vi "PatchCore_DS_Reader_old.vi"(4 "Read Bads?":bool, 5 "Input3D_Custom_Dims":T1, 6 "PreProcessing_Options":T2={"Image Type"=4, "Normalization Type"=enum."Standardize(DS_Stats)", "Interpolation Type"=1} {"Interpolation Type" items=["Zero Order", "Bi-Linear", "Quadratic", "Cubic Spline"]; "Image Type" items=["Grayscale (U8)", "Grayscale (I16)", "Grayscale (SGL)", "Complex (CSG)", "RGB (U32)", "HSL (U32)", "RGB (U64)", "Grayscale (U16)"]}, 7 "Dataset_Stats":T8={"means"={"R"=0.30100304, "G"=0.3015279, "B"=0.32350188}, "vars"={"R"=0.30371806, "G"=0.30376178, "B"=0.2861995}, "DS_Size"=0} {"vars"."R" format="%#_3g"; "vars"."G" format="%#_3g"; "vars"."B" format="%#_3g"; "means"."R" format="%#_3g"; "means"."G" format="%#_3g"; "means"."B" format="%#_3g"}, 8 "error in":errorcluster, 9 "GT Mask Folder Path":path, 10 "Bad Image File Paths":path[](array[path]), 11 "Good Image File Paths":path[](array[path])) -> (0 "error out":errorcluster, 1 "Image Out":sgl[][][][](array[numeric]), 3 "Dataset":T5)   [LabVIEW 2024]
uses:
  <vilib>/Ngene/Deep Learning Toolkit/Toolkit/NN_Data/API/NN_Dims(C,H,W).ctl
  <vilib>/Ngene/Deep Learning Toolkit/Toolkit/Deep_Learning_Toolkit_by_Ngene.lvlib
  <vilib>/Ngene/Deep Learning Toolkit/Toolkit/NN_Data/Controls/DataRef_Types/4D/NN_Data_ref(4D_SGL).ctl
  <vilib>/Ngene/Deep Learning Toolkit/Toolkit/NN_Data/API/DataSet/DataSet_Types/NN_DataSet(In3D_Out3D).ctl
  Tests/Controls/NNPC_DataSets_Good_Bad(In3D_Out3D).ctl
  DeepLTK_Anomaly_Detection_Addon/API/Controls/Image_Stats_RGB.ctl
  DeepLTK_Anomaly_Detection_Addon/API/Controls/NNPC_DS_Stats.ctl
  Tests/Controls/Normalization_Type.ctl
  DeepLTK_Anomaly_Detection_Addon/API/Controls/NNPC_PreProcessing_Options.ctl
panel:
  in  "Good Unique Labels":string[](array[string])
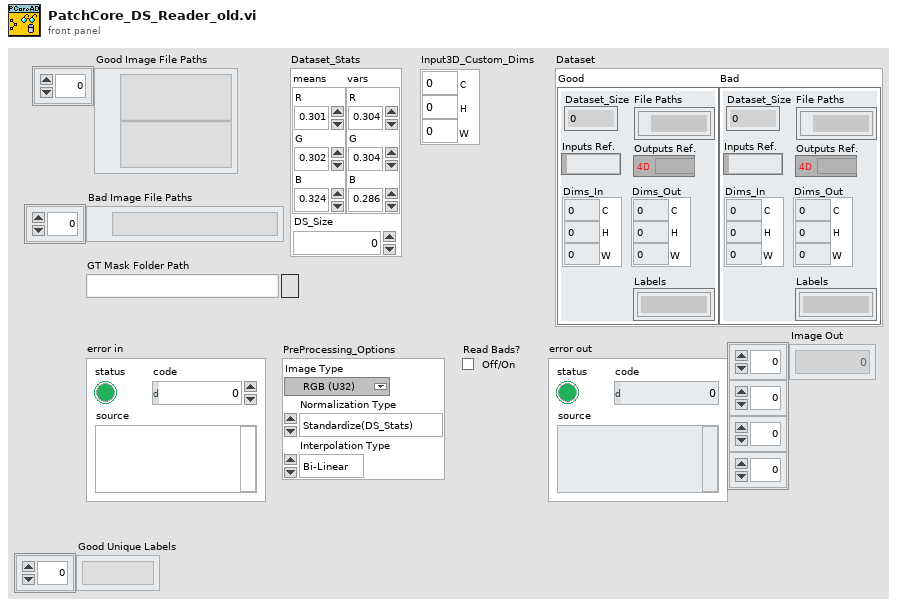
[diagram p1: front panel]
types:
  T1 = typedef "Deep_Learning_Toolkit_by_Ngene.lvlib/NN_Dims(C,H,W).ctl" = cluster{"C":i32, "H":i32, "W":i32}
  T2 = typedef "ImRead_PreProcessing_Options.ctl" = cluster{"Image Type":T3, "Normalization Type":T4, "Interpolation Type":u32}
  T3 = typedef "Image Type" = u32
  T4 = typedef "Normalization_Type.ctl" = enum16{"Standardize(DS_Stats)", "Standardize(Image_Stats)"}
  T5 = typedef "NNPC_DataSets_Good_Bad(In3D_Out3D).ctl" = cluster{"Good":T6, "Bad":T6}
  T6 = typedef "Deep_Learning_Toolkit_by_Ngene.lvlib/NN_DataSet(In3D_Out3D).ctl" = cluster{"Dataset_Size":i32, "Dims_In":T1, "Labels":string[], "File Paths":path[], "Outputs Ref.":T7, "Inputs Ref.":variant, "Dims_Out":T1}
  T7 = typedef "Deep_Learning_Toolkit_by_Ngene.lvlib/NN_Data_ref(4D_SGL).ctl" = refnum<data-value>
  T8 = typedef "NNPC_DS_Stats.ctl" = cluster{"means":T9, "vars":T9, "DS_Size":i32}
  T9 = typedef "Image_Stats_RGB.ctl" = cluster{"R":sgl, "G":sgl, "B":sgl}
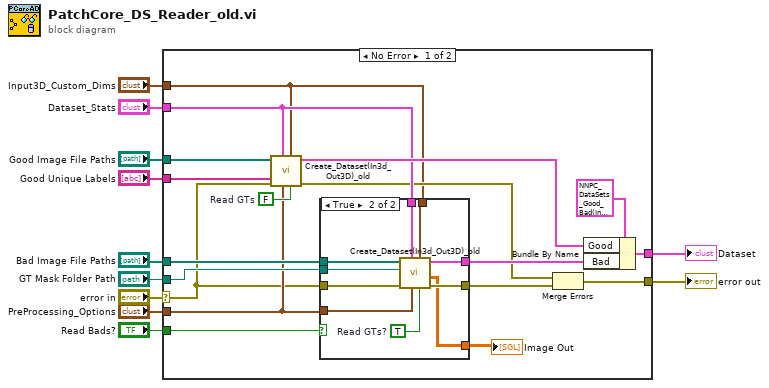
[diagram p0: block diagram]
diagram:
  n1 = case shown="No Error" "error in" {
    selector: "error in" -> [w15 w41]
    tunnel: "Good Image File Paths" -> [w29 _]
    tunnel: [w27 _] -> w10
    tunnel: [w25 w41] -> w9
    tunnel: "Good Unique Labels" -> [w24 _]
    tunnel: "GT Mask Folder Path" -> [w23 _]
    tunnel: "Bad Image File Paths" -> [w22 _]
    tunnel: "Dataset_Stats" -> [w21 _]
    tunnel: "Read Bads?" -> [w18 _]
    tunnel: "PreProcessing_Options" -> [w17 _]
    tunnel: "Input3D_Custom_Dims" -> [w14 _]
    frame No Error {
      w19 = FALSE  # Read GTs
      n2 = call "Create_Dataset(In3d_Out3D)_old.vi"("Read GTs?"=w19, "Input3D_Custom_Dims"=w14, "PreProcessing_Options"=w17, "Dataset_Stats"=w21, "error in (no error)"=w15, "Good Unique Labels"=w24, "Image File Paths"=w29) -> ("error out"=w16:errorcluster, "Dataset(In3D_Out3D)"=w28:T6)  [unwired: 2 in, 1 out]
      n3 = case shown="True" w18 {
        tunnel: [w30 w40] -> w26
        tunnel: w23 -> [_ w39]
        tunnel: w22 -> [_ w38]
        tunnel: w21 -> [_ w37]
        tunnel: [_ w36] -> w20
        tunnel: w17 -> [_ w35]
        tunnel: w15 -> [w30 w34]
        tunnel: w14 -> [_ w32]
        tunnel: [_ w31] -> w12
        frame False {
        }
        frame True {
          w33 = TRUE  # Read GTs?
          n4 = call "Create_Dataset(In3d_Out3D)_old.vi"("Read GTs?"=w33, "Input3D_Custom_Dims"=w32, "PreProcessing_Options"=w35, "Dataset_Stats"=w37, "error in (no error)"=w34, "GT Folder Path"=w39, "Image File Paths"=w38) -> ("error out"=w40:errorcluster, "Image Out"=w31:sgl[][][][], "Dataset(In3D_Out3D)"=w36:T6)  [unwired: 2 in]
        }
      }
      "Image Out" <- w12
      n5 = Merge Errors(w16, w26) -> (w25:errorcluster)
      n6 = Bundle By Name(cluster=T5 {"Good"={"Dataset_Size"=0, "Dims_In"={"C"=0, "H"=0, "W"=0}, "Labels"=[], "File Paths"=[], "Outputs Ref."=refnum, "Inputs Ref."=variant, "Dims_Out"={"C"=0, "H"=0, "W"=0}}, "Bad"={"Dataset_Size"=0, "Dims_In"={"C"=0, "H"=0, "W"=0}, "Labels"=[], "File Paths"=[], "Outputs Ref."=refnum, "Inputs Ref."=variant, "Dims_Out"={"C"=0, "H"=0, "W"=0}}}, "Good"=w28, "Bad"=w20) -> (w27:T5)
    }
    frame Error {
    }
  }
  "error out" <- w9
  "Dataset" <- w10
